vi "DecodeSerialStringToSensorDataArray.vi"(2 "Serial String Queue in":refnum<queue>, 3 "Sensor Data Queue in":refnum<queue>) -> (0 "Line Received":bool, 1 "Line Reset":bool)   [LabVIEW 2013]
panel:
  out "Sensor Line Buffer":string
  out "current sensor line ASCII":string
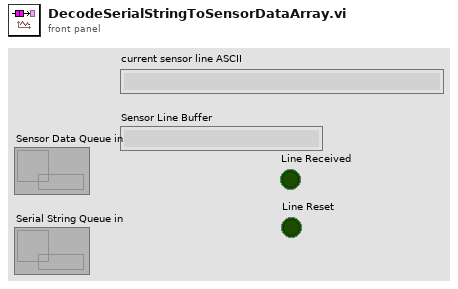
[diagram p1: front panel]
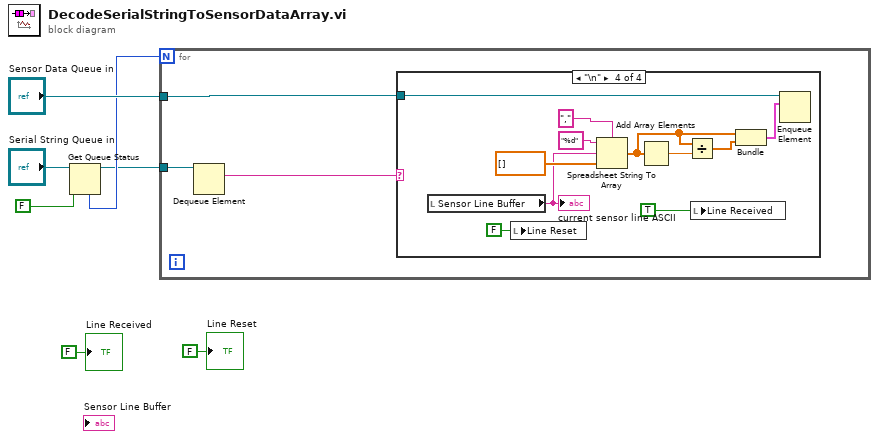
[diagram p0: block diagram]
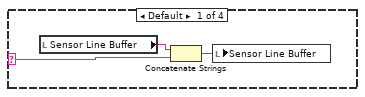
[diagram p2: hidden frame]
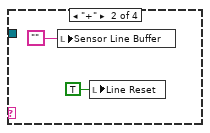
[diagram p3: hidden frame]
diagram:
  n1 = Get Queue Status(queue="Serial String Queue in", return elements? (F)=FALSE) -> (queue out=w1:refnum<queue>, # elements in queue=w3:i32)  [unwired: 1 in, 6 out]
  n2 = for {
    N: w3 -> [_]
    tunnel: "Sensor Data Queue in" -> [w10]
    tunnel: w1 -> [w9]
    n3 = Dequeue Element(queue=w9) -> (element=w8:string)  [unwired: 2 in, 3 out]
    n4 = case shown="\"\\n\"" w8 {
      selector: w8 -> [w13 _ _ _]
      tunnel: w10 -> [_ _ _ w20]
      frame Default {
        n5 = local read "Sensor Line Buffer"() -> (w11:string)
        n6 = Concatenate Strings(w11, w13) -> (w12:string)
        n7 = local write "Sensor Line Buffer"(w12) -> ()
      }
      frame "+" {
        n8 = local write "Sensor Line Buffer"("") -> ()
        n9 = local write "Line Reset"(TRUE ("Line Reset")) -> ()
      }
      frame "\r" {
      }
      frame "\n" {
        n10 = local read "Sensor Line Buffer"() -> (w18:string)
        "current sensor line ASCII" <- w18
        n11 = local write "Line Reset"(FALSE ("Line Reset")) -> ()
        n12 = Spreadsheet String To Array(delimiter (Tab)=",", format string="%d", spreadsheet string=w18, array type (2D Dbl)=dbl[] []) -> (array=w21:dbl[])
        n13 = Add Array Elements(numeric array=w21) -> (sum=w23:dbl)
        n14 = Divide(x=w21, y=w23) -> (x/y=w22:dbl[])
        n15 = local write "Line Received"(TRUE ("Line Received")) -> ()
        n16 = Bundle("array type (2D Dbl)"=w21, w22) -> (w19:cluster{"array type (2D Dbl)":dbl[], dbl[]})  [unwired: 1 in]
        n17 = Enqueue Element(queue=w20, element=w19) -> ()  [unwired: 2 in, 3 out]
      }
    }
  }
  "Line Received" <- FALSE ("Line Received")
  "Line Reset" <- FALSE ("Line Reset")
